vi "load string.vi"(10 "Array in":string[](array[string]), 11 "Codice":string) -> (1 "ID bollettino":string[](array[string]), 2 "Numeric":i32, 3 "String command":string)   [LabVIEW 2019]
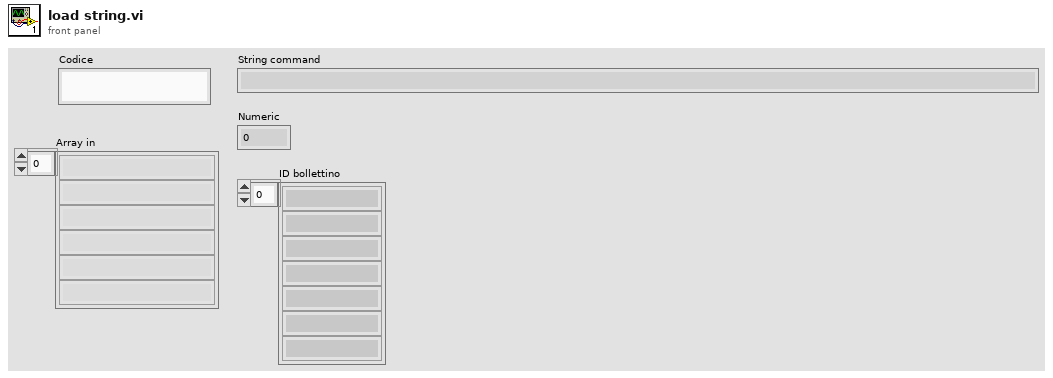
[diagram p1: front panel]
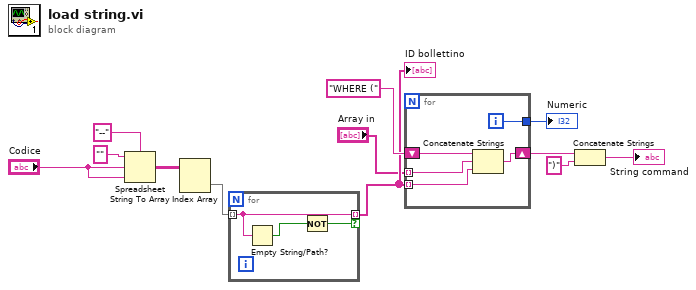
[diagram p0: block diagram]
diagram:
  n1 = Spreadsheet String To Array(delimiter (Tab)="--", format string="", spreadsheet string="Codice", array type (2D Dbl)="Codice") -> (array=w4:string[][])
  n2 = Index Array(array=w4) -> (element=w3:string[])  [unwired: 2 in]
  n3 = for {
    tunnel: w3 -> [w15] mode=indexing
    tunnel: [w15] -> w2 mode=indexing if=w13
    n4 = Empty String/Path?(string/path=w15) -> (empty?=w14:bool)
    n5 = Not(x=w14) -> (.not. x?=w13:bool)
  }
  "ID bollettino" <- w2
  n6 = for {
    tunnel: "Array in" -> [w16] mode=indexing
    tunnel: w2 -> [w17] mode=indexing
    shift-right: [w19] -> w8
    shift-left: "WHERE (" ("condition") -> [w20]
    tunnel: [w18] -> w11
    i -> [w18]
    n7 = Concatenate Strings(w20, w16, w17) -> (w19:string)
  }
  "Numeric" <- w11
  n8 = Concatenate Strings(w8, ")" ("string")) -> (→"String command":string)
